vi "kvCanReadSyncSpecific.vi"(2 "error in (no error)":errorcluster, 3 "Timeout":u32, 4 "Message Id":i32, 5 "Channel Handle (input only)":i32) -> (0 "error out":errorcluster, 1 "Channel Handle (ouput only)":i32)   [LabVIEW 2022 SP3]
doc: "Waits until the receive queue contains a message with the specified id, or a timeout occurs."
uses:
  canlib32.dll
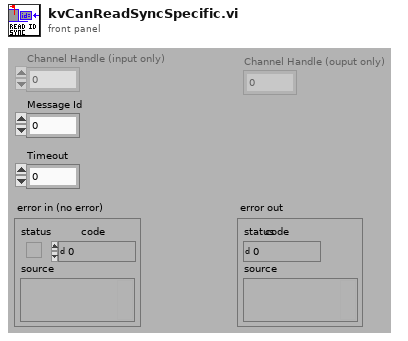
[diagram p1: front panel]
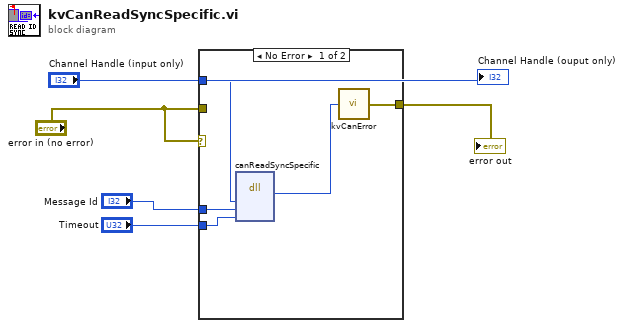
[diagram p0: block diagram]
diagram:
  n1 = case shown="No Error" "error in (no error)" {
    tunnel: "error in (no error)" -> [_ w11]
    tunnel: "Channel Handle (input only)" -> [w9 _]
    tunnel: [w8 w11] -> w3
    tunnel: "Message Id" -> [w7 _]
    tunnel: "Timeout" -> [w6 _]
    frame No Error {
      n2 = dll-call lib="canlib32.dll" fn="canReadSyncSpecific" label="Call CanReadSyncSpecific"("channelHandle"=w9, "id"=w7, "timeout"=w6) -> (w10:i32)  [unwired: 6 in, 2 out]
      n3 = call "kvCanError.vi"("error code"=w10) -> ("error out"=w8:errorcluster)
    }
    frame Error {
    }
  }
  "error out" <- w3
  "Channel Handle (ouput only)" <- "Channel Handle (input only)"
